vi "Sequence Read.vi"(8 "error in (no error)":errorcluster, 11 "SimSyA in":refnum<class "SimSyA.lvclass">) -> (0 "error out":errorcluster, 1 "Control Data":T3, 2 "Acquisition Data":T1, 3 "SimSyA out":refnum<class "SimSyA.lvclass">)   [LabVIEW 2014, in "SimSyA.lvlib" / "SimSyA.lvclass"]
uses:
  SimSyA.lvclass
  DriverMasterSync/build/DriverMasterSync.lvlibp/APIs/Data Queue/Control Data Cluster.ctl
  DriverMasterSync/build/DriverMasterSync.lvlibp/APIs/Data Queue/Acquisition Data Cluster.ctl
  DriverMasterSync/build/DriverMasterSync.lvlibp/APIs/Data Queue/Acquisition Data 1 Sample Cluster.ctl
  SimSyA.lvclass/SimSyA.ctl
  DriverMasterSync/build/DriverMasterSync.lvlibp/Modules/HAL/DriverMasterSync/DriverMasterSyncClass/DriverMasterSync.lvclass
  SimSyA.lvlib
  DriverMasterSync/build/DriverMasterSync.lvlibp/APIs/Data Queue/WINFAS 2 Data Queue.lvlib
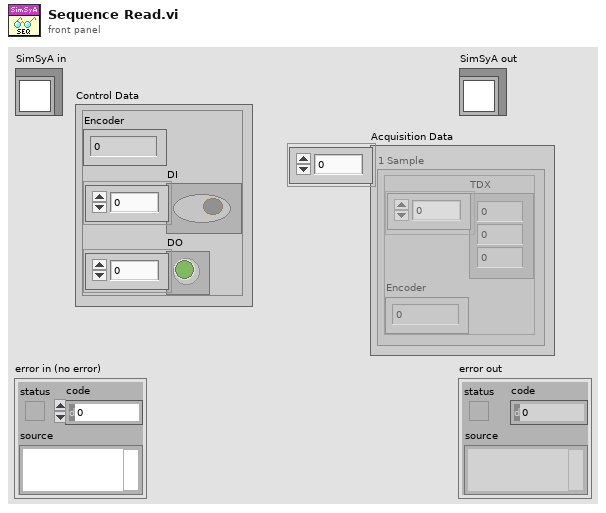
[diagram p1: front panel]
types:
  T1 = typedef "DriverMasterSync.lvlibp/WINFAS 2 Data Queue.lvlib/Acquisition Data Cluster.ctl" = T2[]
  T2 = typedef "DriverMasterSync.lvlibp/WINFAS 2 Data Queue.lvlib/Acquisition Data 1 Sample Cluster.ctl" = cluster{"TDX":sgl[], "Encoder":sgl}
  T3 = typedef "DriverMasterSync.lvlibp/WINFAS 2 Data Queue.lvlib/Control Data Cluster.ctl" = cluster{"Encoder":sgl, "DI":bool[], "DO":bool[]}
  T4 = cluster{"TDX":sgl[], "Encoder":i32, "DI Counter":u32, "DO Mask":u32}
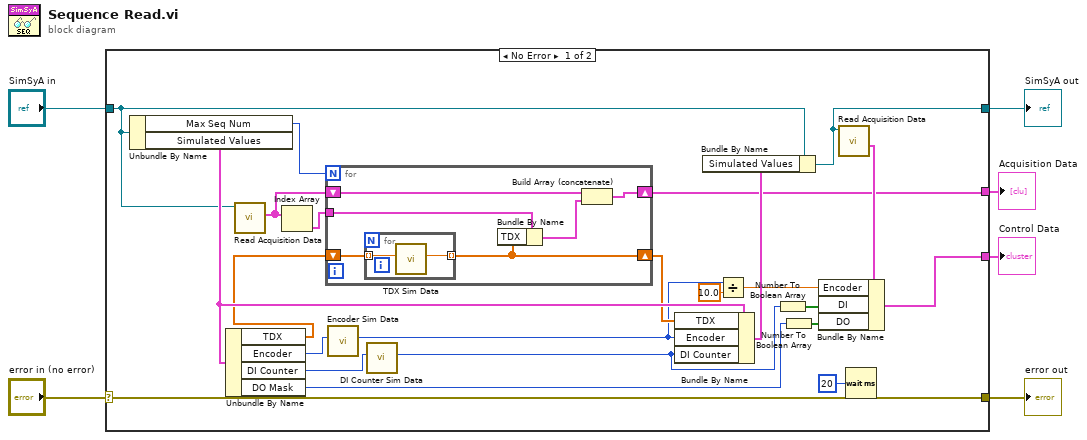
[diagram p0: block diagram]
diagram:
  n1 = case shown="No Error" "error in (no error)" {
    selector: "error in (no error)" -> [w29 w39]
    tunnel: [w29 w39] -> w5
    tunnel: [w18 w38] -> w3
    tunnel: "SimSyA in" -> [w10 w38]
    tunnel: [w14 _] -> w2
    tunnel: [w11 _] -> w1
    frame No Error {
      n2 = Unbundle By Name(w10) -> ("Max Seq Num"=w15:u64, "Simulated Values"=w25:T4)
      n3 = Unbundle By Name(w25) -> ("TDX"=w16:sgl[], "Encoder"=w21:i32, "DI Counter"=w22:u32, "DO Mask"=w26:u32)
      n4 = call "Read Acquisition Data.vi"("DriverMasterSync in"=w10) -> ("Acquisition Data"=w12:T1)  [unwired: 7 in, 3 out]
      n5 = Index Array(array=w12) -> (element=w13:T2)  [unwired: 1 in]
      n6 = for {
        N: w15 -> [_]
        shift-right: [w34] -> w17
        shift-left: w16 -> [w35]
        tunnel: w13 -> [w33]
        shift-right: [w31] -> w11
        shift-left: w12 -> [w30]
        n7 = for {
          tunnel: w35 -> [w37] mode=indexing
          tunnel: [w36] -> w34 mode=indexing
          n8 = call "TDX Sim Data.vi"("TDX in"=w37) -> ("TDX out"=w36:sgl)  [unwired: 10 in]
        }
        n9 = Bundle By Name(cluster=w33, "TDX"=w34) -> (w32:T2)
        n10 = Build Array (concatenate)(w30, w32) -> (w31:T1)
      }
      n11 = call "Encoder Sim Data.vi"("Encoder in"=w21) -> ("Encoder out"=w8:i32)  [unwired: 10 in]
      n12 = call "DI Counter Sim Data.vi"("DI Counter in"=w22) -> ("DI Counter out"=w19:u32)  [unwired: 10 in]
      n13 = Bundle By Name(cluster=w25, "TDX"=w17, "Encoder"=w8, "DI Counter"=w19) -> (w24:T4)
      n14 = Bundle By Name(cluster=w10, "Simulated Values"=w24) -> (w18:refnum<class "SimSyA.lvclass">)
      n15 = Divide(x=w8, y=10.0) -> (x/y=w7:dbl)
      n16 = Number To Boolean Array(number=w19) -> (Boolean array=w20:bool[])
      n17 = Number To Boolean Array(number=w26) -> (Boolean array=w27:bool[])
      n18 = call "Read Acquisition Data.vi"("DriverMasterSync in"=w18) -> ("Control Data"=w28:T3)  [unwired: 7 in, 3 out]
      n19 = Bundle By Name(cluster=w28, "Encoder"=w7, "DI"=w20, "DO"=w27) -> (w14:T3)
      n20 = Wait (ms)(milliseconds to wait=u32 20) -> ()  [unwired: 1 out]
    }
    frame Error {
    }
  }
  "error out" <- w5
  "SimSyA out" <- w3
  "Control Data" <- w2
  "Acquisition Data" <- w1
